vi "CH2_Comm_TCPIP_NEW.vi"() -> ()   [LabVIEW 2018]
uses:
  RxTx/RxTx.lvclass
panel:
  in  "IP 2":string="200.131.64.49"
  in  "stop":bool
  out "error out 5":errorcluster
  out "error out 4":errorcluster
  out "error out 3":errorcluster
  out "error out 2":errorcluster
  in  "RxTx.lvclass 2":refnum<class "RxTx.lvclass">
  in  "Channel":u16=2
  # "Channel 1 - TCPIP Communication"
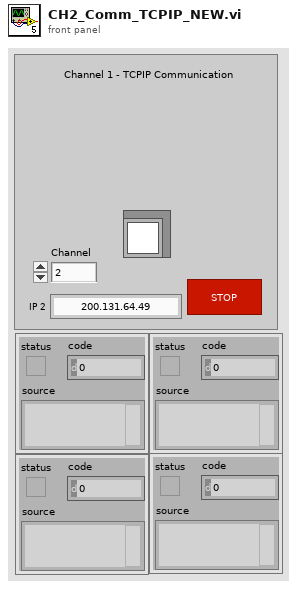
[diagram p1: front panel]
types:
  T1 = enum16{"Standard", "Buffered", "CRLF", "Immediate"}
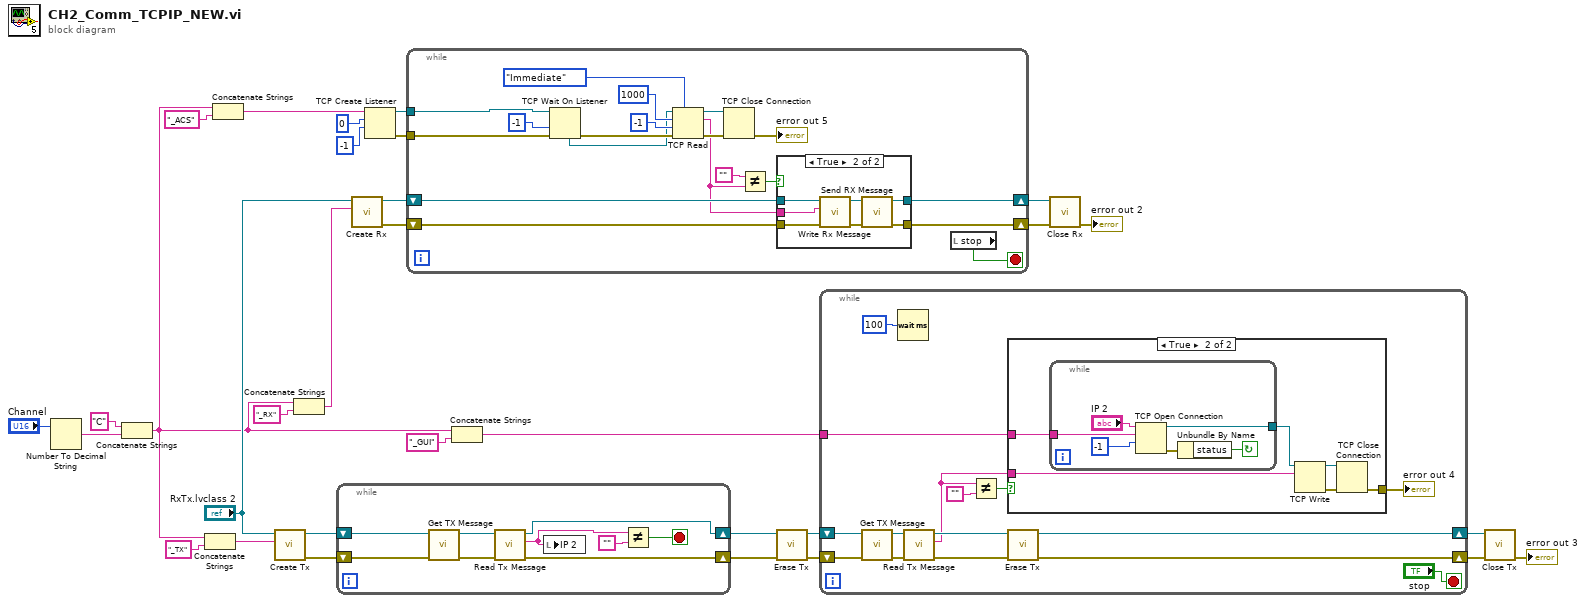
[diagram p0: block diagram]
diagram:
  n1 = Number To Decimal String(number="Channel") -> (decimal integer string=w28:string)  [unwired: 1 in]
  n2 = Concatenate Strings("C", w28) -> (w7:string)
  n3 = Concatenate Strings(w7, "_TX" ("Reader Name")) -> (w22:string)
  n4 = Concatenate Strings(w7, "_ACS" ("Reader Name")) -> (w12:string)
  n5 = call "Create Tx.vi"("Writer Name"=w22, "RxTx in"="RxTx.lvclass 2") -> ("error out"=w5:errorcluster, "RxTx out"=w6:refnum<class "RxTx.lvclass">)  [unwired: 8 in]
  n6 = Concatenate Strings(w7, "_RX" ("Reader Name")) -> (w31:string)
  n7 = while {
    shift-right: [w38] -> w4
    shift-left: w6 -> [w40]
    shift-right: [w37] -> w1
    shift-left: w5 -> [w35]
    stop <- w33 stop-if-true
    n8 = call "Get TX Message.vi"("error in (no error)"=w35, "RxTx in"=w40) -> ("error out"=w36:errorcluster, "RxTx out"=w39:refnum<class "RxTx.lvclass">)  [unwired: 8 in]
    n9 = call "Read Tx Message.vi"("error in (no error)"=w36, "RxTx in"=w39) -> ("error out"=w37:errorcluster, "Tx Message"=w32:string, "RxTx out"=w38:refnum<class "RxTx.lvclass">)  [unwired: 7 in]
    n10 = local write "IP 2"(w32) -> ()
    n11 = Not Equal?(x=w32, y="") -> (x != y?=w33:bool)
  }
  n12 = call "Create Rx.vi"("Reader Name"=w31, "RxTx in"="RxTx.lvclass 2") -> ("error out"=w26:errorcluster, "RxTx out"=w27:refnum<class "RxTx.lvclass">)  [unwired: 8 in]
  n13 = TCP Create Listener(9:-1 ("timeout ms (25000)"), 10:u16 0 ("port"), 11:w12) -> (0:w9:errorcluster, 3:w10:refnum<k5>)  [unwired: 2 in, 1 out]
  n14 = while {
    shift-right: [w54] -> w24
    shift-left: w26 -> [w59]
    shift-right: [w55] -> w25
    shift-left: w27 -> [w58]
    tunnel: w10 -> [w52]
    tunnel: w9 -> [w43]
    stop <- w53 stop-if-true
    n15 = TCP Wait On Listener(8:w43, 9:-1 ("timeout ms (wait forever: -1)"), 11:w52) -> (0:w47:errorcluster, 4:w42:refnum<k5>)  [unwired: 1 in, 3 out]
    n16 = TCP Read(connection ID=w42, bytes to read=1000, error in (no error)=w47, 7:T1."Immediate" ("mode (standard)"), 9:-1 ("timeout ms (25000)")) -> (connection ID out=w45:refnum<k5>, data out=w41:string, error out=w44:errorcluster)
    n17 = TCP Close Connection(connection ID=w45, error in (no error)=w44) -> (error out=→"error out 5":errorcluster)  [unwired: 1 in, 1 out]
    n18 = Not Equal?(x="", y=w41) -> (x != y?=w56:bool)
    n19 = case shown="True" w56 {
      tunnel: w59 -> [w60 w66]
      tunnel: w58 -> [w61 w65]
      tunnel: [w61 w64] -> w55
      tunnel: [w60 w63] -> w54
      tunnel: w41 -> [_ w62]
      frame False {
      }
      frame True {
        n20 = call "Write Rx Message.vi"("error in (no error)"=w66, "Rx Message"=w62, "RxTx in"=w65) -> ("error out"=w67:errorcluster, "RxTx out"=w68:refnum<class "RxTx.lvclass">)  [unwired: 7 in]
        n21 = call "Send RX Message.vi"("error in (no error)"=w67, "RxTx in"=w68) -> ("error out"=w63:errorcluster, "RxTx out"=w64:refnum<class "RxTx.lvclass">)  [unwired: 8 in]
      }
    }
    n22 = local read "stop"() -> (w53:bool)
  }
  n23 = Concatenate Strings(w7, "_GUI" ("Reader Name")) -> (w13:string)
  n24 = call "Erase Tx.vi"("error in (no error)"=w1, "RxTx in"=w4) -> ("error out"=w2:errorcluster, "RxTx out"=w3:refnum<class "RxTx.lvclass">)  [unwired: 8 in]
  n25 = while {
    shift-right: [w83] -> w20
    shift-left: w3 -> [w76]
    shift-right: [w82] -> w19
    shift-left: w2 -> [w75]
    tunnel: w13 -> [w69]
    stop <- "stop" stop-if-true
    n26 = call "Get TX Message.vi"("error in (no error)"=w75, "RxTx in"=w76) -> ("error out"=w81:errorcluster, "RxTx out"=w77:refnum<class "RxTx.lvclass">)  [unwired: 8 in]
    n27 = Wait (ms)(milliseconds to wait=u32 100) -> ()  [unwired: 1 out]
    n28 = call "Read Tx Message.vi"("error in (no error)"=w81, "RxTx in"=w77) -> ("error out"=w78:errorcluster, "Tx Message"=w70:string, "RxTx out"=w79:refnum<class "RxTx.lvclass">)  [unwired: 7 in]
    n29 = Not Equal?(x=w70, y="") -> (x != y?=w74:bool)
    n30 = case shown="True" w74 {
      tunnel: w70 -> [_ w88]
      tunnel: [_ w84] -> w73
      tunnel: w69 -> [_ w89]
      frame False {
      }
      frame True {
        n31 = while {
          tunnel: w89 -> [w94]
          tunnel: [w91] -> w87
          stop <- w95 continue-if-true
          n32 = TCP Open Connection(address="IP 2", remote port or service name=w94, timeout ms (60000)=-1 ("timeout")) -> (connection ID=w91:refnum<k5>, error out=w93:errorcluster)  [unwired: 2 in]
          n33 = Unbundle By Name(w93) -> ("status"=w95:bool)
        }
        n34 = TCP Write(connection ID=w87, data in=w88) -> (connection ID out=w85:refnum<k5>, error out=w86:errorcluster)  [unwired: 2 in, 1 out]
        n35 = TCP Close Connection(connection ID=w85, error in (no error)=w86) -> (error out=w84:errorcluster)  [unwired: 1 in, 1 out]
      }
    }
    "error out 4" <- w73
    n36 = call "Erase Tx.vi"("error in (no error)"=w78, "RxTx in"=w79) -> ("error out"=w82:errorcluster, "RxTx out"=w83:refnum<class "RxTx.lvclass">)  [unwired: 8 in]
  }
  n37 = call "Close Rx.vi"("error in (no error)"=w24, "RxTx in"=w25) -> ("error out"=→"error out 2":errorcluster)  [unwired: 8 in, 1 out]
  n38 = call "Close Tx.vi"("error in (no error)"=w19, "RxTx in"=w20) -> ("error out"=→"error out 3":errorcluster)  [unwired: 8 in, 1 out]
